vi "Build Status Message.vi"(6 "Start Time":timestamp, 8 "Step Repeat":i32, 9 "Macro Repeat":i32, 10 "Step":i32, 11 "Macro":T1) -> (3 "Status":string)   [LabVIEW 2020, in "MacroAssert.lvlib"]
doc: "Builds a status message to be displayed to the user, using the given inputs."
uses:
  MacroAssert.lvlib
  CTLs/Macro Cluster V3.ctl
  CTLs/Macro Config V3.ctl
  CTLs/Step V3.ctl
  CTLs/Step Type V3.ctl
  <userlib>/_OpenG.lib/array/array.llb/Filter 1D Array with Scalar (String)__ogtk.vi
  <userlib>/_OpenG.lib/array/array.llb/openg_array.lvlib
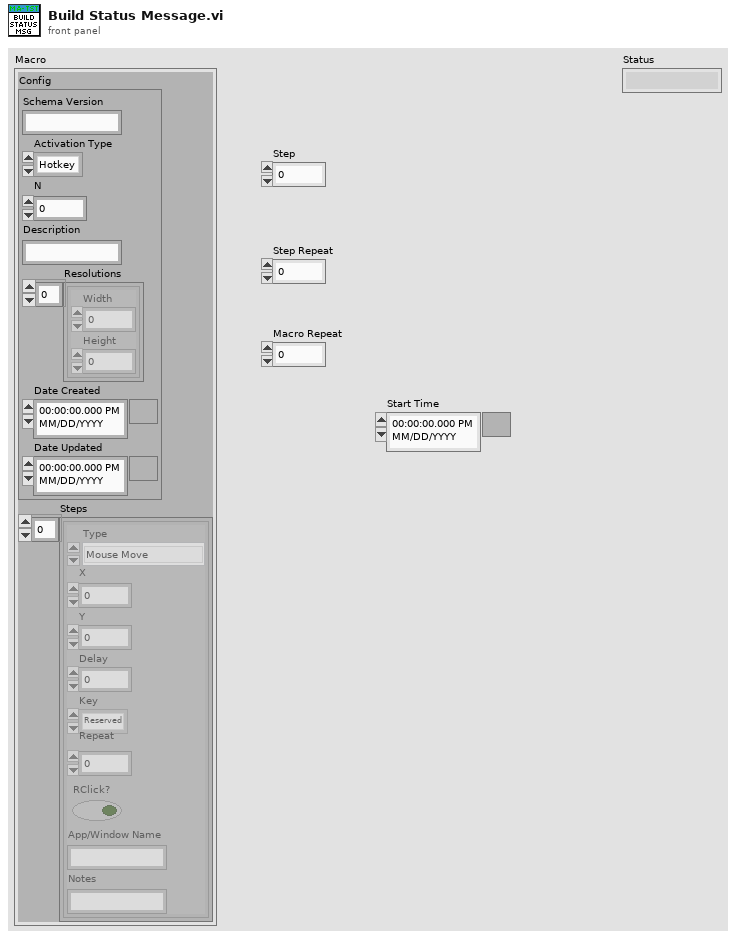
[diagram p1: front panel]
types:
  T1 = typedef "MacroAssert.lvlib/Macro Cluster V3.ctl" = cluster{"Config":T2, "Steps":T3[]}
  T2 = typedef "MacroAssert.lvlib/Macro Config V3.ctl" = cluster{"Schema Version":string, "Activation Type":enum32{"Hotkey", "Automatic"}, "N":i32, "Description":string, "Resolutions":cluster{"Width":i16, "Height":i16}[], "Date Created":timestamp, "Date Updated":timestamp}
  T3 = typedef "MacroAssert.lvlib/Step V3.ctl" = cluster{"Type":T4, "X":i32, "Y":i32, "Delay":i32, "Key":u8, "Repeat":i32, "RClick?":bool, "App/Window Name":string, "Notes":string}
  T4 = typedef "MacroAssert.lvlib/Step Type V3.ctl" = enum16{"Mouse Move", "Mouse Click", "Key Press", "Wait", "Mouse Down", "Mouse Up", "Key Down", "Key Up", "Run Application", "Maximize Window", "Restore Window", "Minimize Window", "Close Window", "Bring Window to Front", "Send Window to Back"}
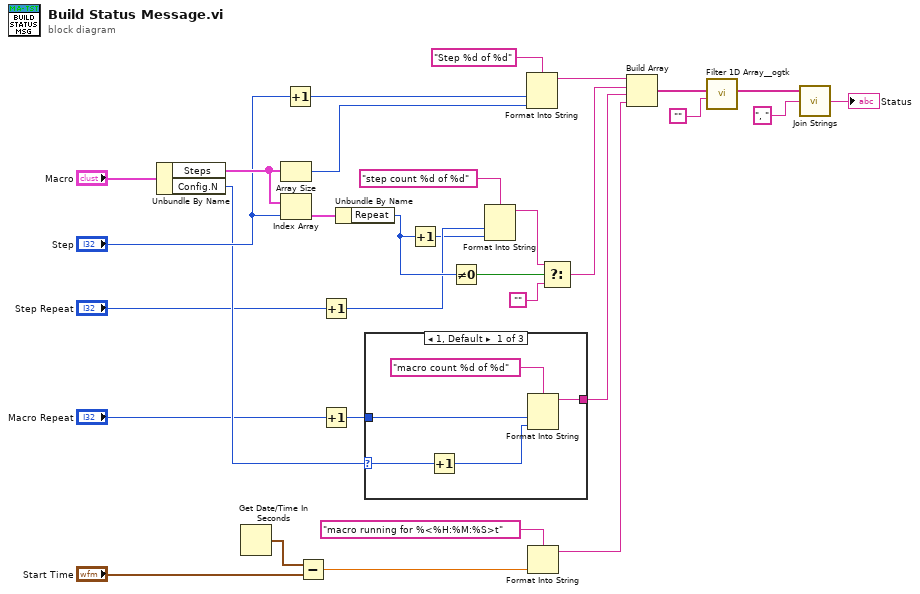
[diagram p0: block diagram]
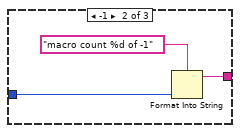
[diagram p2: hidden frame]
diagram:
  n1 = Unbundle By Name("Macro") -> ("Steps"=w29:T3[], "Config.N"=w16:i32)
  n2 = Get Date/Time In Seconds() -> (seconds since 1Jan1904=w14:timestamp)
  n3 = Array Size(array=w29) -> (size(s)=w25:i32)
  n4 = Index Array(array=w29, index="Step") -> (element=w31:T3)
  n5 = Increment(x="Step") -> (x+1=w23:i32)
  n6 = Subtract(x=w14, y="Start Time") -> (x-y=w12:dbl)
  n7 = Increment(x="Step Repeat") -> (x+1=w21:i32)
  n8 = Increment(x="Macro Repeat") -> (x+1=w17:i32)
  n9 = Unbundle By Name(w31) -> ("Repeat"=w22:i32)
  n10 = case shown="1, Default" w16 {
    selector: w16 -> [w33 _ _]
    tunnel: w17 -> [w35 w38 _]
    tunnel: [w34 w37 _] -> w9
    frame 1, Default {
      n11 = Increment(x=w33) -> (x+1=w32:i32)
      n12 = Format Into String(format string="macro count %d of %d", w35, w32) -> (resulting string=w34:string)  [unwired: 2 in, 1 out]
    }
    frame -1 {
      n13 = Format Into String(format string="macro count %d of -1", w38) -> (resulting string=w37:string)  [unwired: 2 in, 1 out]
    }
    frame 0 {
    }
  }
  n14 = Increment(x=w22) -> (x+1=w20:i32)
  n15 = Not Equal To 0?(x=w22) -> (x != 0?=w27:bool)
  n16 = Format Into String(format string="step count %d of %d", w21, w20) -> (resulting string=w19:string)  [unwired: 2 in, 1 out]
  n17 = Format Into String(format string="Step %d of %d", w23, w25) -> (resulting string=w11:string)  [unwired: 2 in, 1 out]
  n18 = Format Into String(format string="macro running for %<%H:%M:%S>t", w12) -> (resulting string=w8:string)  [unwired: 2 in, 1 out]
  n19 = Select(t=w19, s=w27, f="") -> (s? t:f=w10:string)
  n20 = Build Array(w11, w10, w9, w8) -> (w7:string[])
  n21 = call-poly <userlib>:"Filter 1D Array__ogtk.vi"("items to filter"="", "array"=w7) -> ("filtered array"=w5:string[])  [unwired: 4 in, 1 out]
  n22 = call <vilib>:"Join Strings.vi"("Separator (,)"=", ", "Strings In"=w5) -> ("String"=→"Status":string)  [unwired: 1 in]
